vi "Call Get Private Event Loops.vi"(8 "error in":errorcluster, 11 "Library":refnum<class "Library.lvclass">) -> (0 "error out":errorcluster, 2 "Consuming Event Structures":refnum<vi>[](array[refnum]), 3 "Consuming Loop Names":string[](array[string]))   [LabVIEW 2020, in "Panther Dashboard.lvlib" / "Library.lvclass"]
uses:
  Library.lvclass
  Library.lvclass/Library.ctl
  Read Library Ref.vi
  Panther Dashboard/Panther Dashboard.lvlib
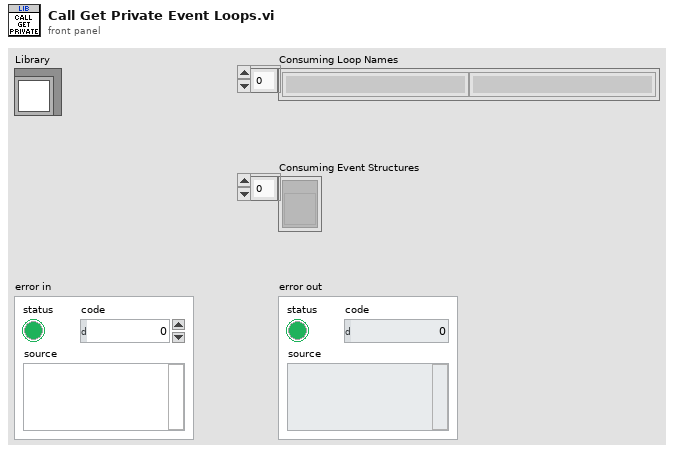
[diagram p1: front panel]
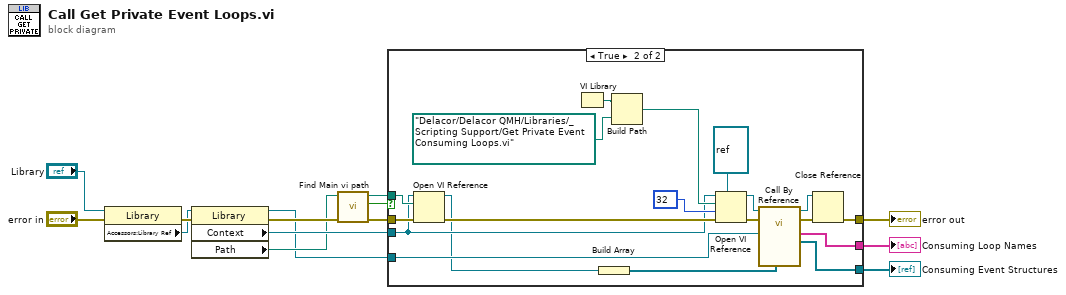
[diagram p0: block diagram]
diagram:
  n1 = property class="Library"(reference="Library", error in="error in") -> (error out=w13:errorcluster, "Accessors:Library Ref"=w8:refnum<vi>)  [unwired: 1 out]
  n2 = property class="Library"(reference=w8, error in=w13) -> (reference out=w2:refnum<vi>, error out=w11:errorcluster, "Context"=w9:refnum<vi>, "Path"=w5:path)
  n3 = call "Find Main vi path.vi"("error in"=w11, "Library Path"=w5) -> ("error out"=w10:errorcluster, "Main.vi Found?"=w4:bool, "Main vi Path"=w3:path)  [unwired: 7 in]
  n4 = case shown="True" w4 {
    tunnel: w9 -> [_ w18]
    tunnel: [w15 w32] -> w12
    tunnel: w2 -> [_ w22]
    tunnel: [_ w21] -> w7
    tunnel: [_ w20] -> w6
    tunnel: w10 -> [w15 w31]
    tunnel: w3 -> [_ w19]
    frame False {
    }
    frame True {
      n5 = Open VI Reference(application reference (local)=w18, vi path=w19, error in (no error)=w31) -> (vi reference=w17:refnum<vi>, error out=w30:errorcluster)  [unwired: 3 in]
      n6 = VI Library() -> (path=w23:path)
      n7 = Build Array(w17) -> (w16:refnum<vi>[])
      n8 = Build Path(base path=w23, name or relative path=path "Delacor/Delacor QMH/Libraries/_Scripting Support/Get Private Event Consuming Loops.vi") -> (appended path=w27:path)
      n9 = Open VI Reference(type specifier VI Refnum (for type only)=refnum<vi> refnum, application reference (local)=w18, vi path=w27, options=32, error in (no error)=w30) -> (vi reference=w29:refnum<vi>, error out=w33:errorcluster)  [unwired: 1 in]
      n10 = call-by-ref "?"(reference=w29, error in=w33, "Cached Main VIs in"=w16, "Library"=w22) -> (reference out=w28:refnum<vi>, error out=w34:errorcluster, "Consuming Event Structures"=w21:refnum<vi>[], "Consuming Loop Names"=w20:string[])  [unwired: 6 in, 2 out]
      n11 = Close Reference(reference=w28, error in (no error)=w34) -> (error out=w32:errorcluster)
    }
  }
  "error out" <- w12
  "Consuming Event Structures" <- w7
  "Consuming Loop Names" <- w6
